vi "Read I32.vi"(8 "error in (no error)":errorcluster, 9 "offset (0)":u64 format="%d bytes", 10 "value in":i32, 11 "Pointer in":refnum<class "Pointer.lvclass">) -> (0 "error out":errorcluster, 1 "offset out":u64 format="%d bytes", 2 "value out":i32, 3 "Pointer out":refnum<class "Pointer.lvclass">)   [LabVIEW 2027, in "Memory Manager.lvlib" / "Pointer.lvclass"]
doc: "Reads <b>value</b> from the address specified by <b>pointer + offset</b>."
uses:
  Pointer.lvclass
  Read (No Check) I32.vi
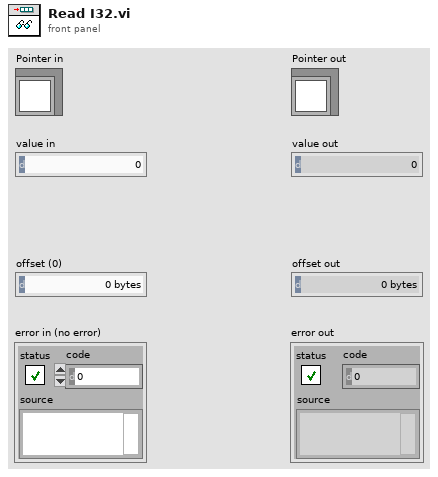
[diagram p1: front panel]
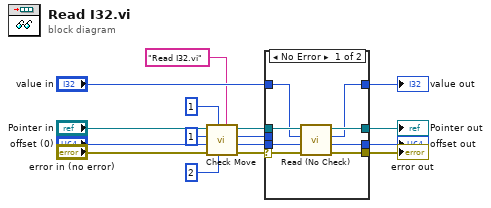
[diagram p0: block diagram]
diagram:
  n1 = call "Check Move.vi"("source vi name"="Read I32.vi", "count power of 2"=u8 2, "buffer count"=u64 1, "error in (no error)"="error in (no error)", "offset (0)"="offset (0)", "move count (-1: rest)"=i64 1, "Pointer in"="Pointer in") -> ("error out"=w10:errorcluster, "offset"=w9:u64, "count"=w8:u64, "Pointer out"=w11:refnum<class "Pointer.lvclass">)  [unwired: 1 in]
  n2 = case shown="No Error" w10 {
    selector: w10 -> [w24 w27]
    tunnel: w11 -> [w22 w26]
    tunnel: w9 -> [w23 w28]
    tunnel: "value in" -> [w17 w25]
    tunnel: [w21 w27] -> w16
    tunnel: [w20 w26] -> w14
    tunnel: [w19 w28] -> w13
    tunnel: [w18 w25] -> w15
    tunnel: w8 -> [_ _]
    frame No Error {
      n3 = call-poly "Read (No Check).vi"("error in (no error)"=w24, "offset (0)"=w23, "value in"=w17, "Pointer in"=w22) -> ("error out"=w21:errorcluster, "offset + size"=w19:u64, "value out"=w18:i32, "Pointer out"=w20:refnum<class "Pointer.lvclass">)  [unwired: 4 in]
    }
    frame Error {
    }
  }
  "error out" <- w16
  "Pointer out" <- w14
  "value out" <- w15
  "offset out" <- w13
